vi "File Page - Get Log File Settings.vi"(7 "File Ctl Refs":T1, 8 "error in (no error)":errorcluster, 11 "Item Ref in":T11 format="%.0x") -> (0 "error out":errorcluster, 3 "Item Ref out":T11 format="%.0x")   [LabVIEW 2015, in "Waveform Data Logger System Explorer.lvlib"]
uses:
  Waveform Data Logger System Explorer.lvlib
  <vilib>/NI Veristand/Custom Device API/Custom Device Item Ref.ctl
  Types/File Ctl Refs.ctl
  Types/File - Spec Ctl Refs.ctl
  Types/File - Wfm Ctl Refs.ctl
  Types/File - Settings Ctl Refs.ctl
  Shared/Classes/Log File Specifications/Log File Specification/File Conflict Operation.ctl
  Types/File - Start Trig Ctl Refs.ctl
  Shared/Types/Start Trigger.ctl
  Shared/Types/Default Trigger.ctl
  Shared/Types/Digital Trigger.ctl
  Shared/Types/Analog Trigger.ctl
  Shared/Types/In Range Trigger.ctl
  Shared/Types/Value Change Trigger.ctl
  Shared/Types/Boolean Trigger.ctl
  Types/Single Node Browser Data.ctl
  <vilib>/NI Veristand/UI Controls/Single Node Browser/Single Node Browser Ref.ctl
  NationalInstruments.VeriStand.SystemStorageUI
  <vilib>/NI Veristand/UI Controls/Single Node Browser/Callback Type.ctl
  <vilib>/NI Veristand/UI Controls/Single Node Browser/Net Event Data.ctl
  <vilib>/NI Veristand/UI Controls/Single Node Browser/Net Event.ctl
  Types/File - Stop Trig Ctl Refs.ctl
  Shared/Types/Stop Trigger.ctl
  Types/File - Advanced Ctl Refs.ctl
  Types/Log Timestamps.ctl
  Shared/Globals/Property Strings.vi
  <vilib>/NI Veristand/Custom Device API/Get Item Property (Boolean).vi
  <vilib>/NI Veristand/Custom Device API/Get Item Property (String).vi
  <vilib>/NI Veristand/Custom Device API/Get Item Property (U16).vi
  <vilib>/NI Veristand/Custom Device API/Get Item Property (Double).vi
  Shared/Waveform Data Logger Shared.lvlib
  <vilib>/NI VeriStand/Custom Device API/Custom Device API.lvlib
  Shared/Classes/Log File Specifications/Log File Specification/Log File Specification.lvclass
  <vilib>/NI VeriStand/UI Controls/Single Node Browser/NI_VS UI Single Node Browser.lvlib
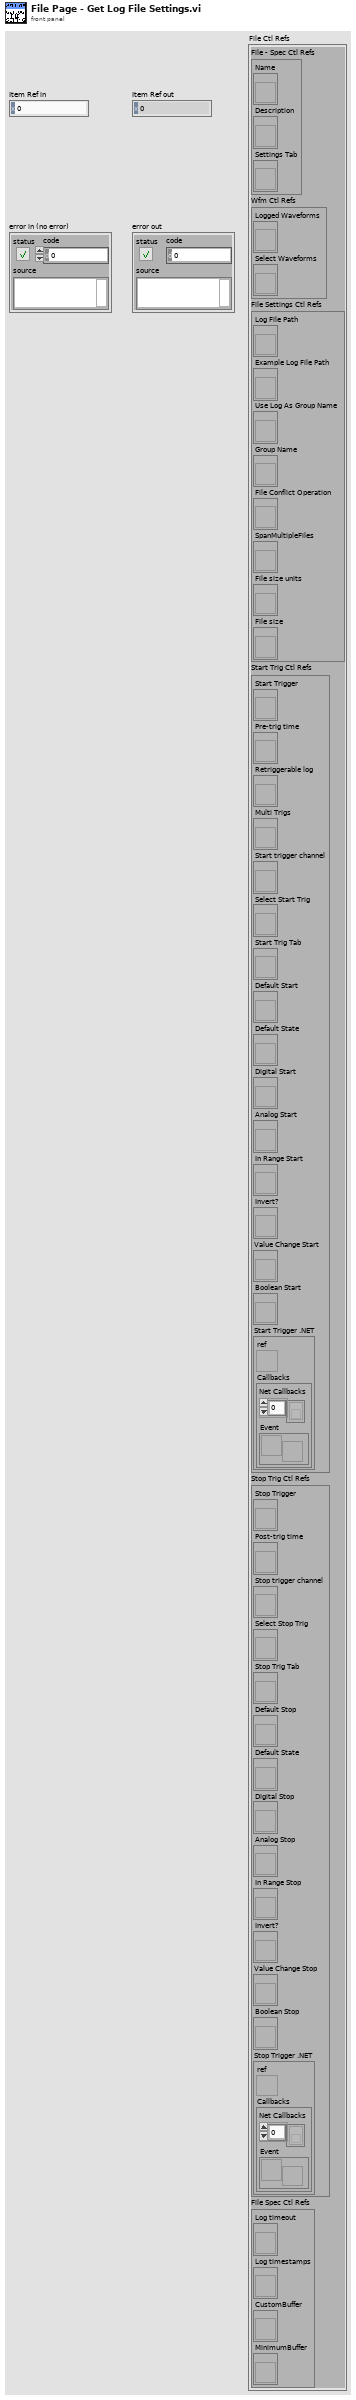
[diagram p1: front panel]
types:
  T1 = typedef "Waveform Data Logger System Explorer.lvlib/File Ctl Refs.ctl" = cluster{"File Spec Ctl Refs":T2, "Wfm Ctl Refs":T3, "File Settings Ctl Refs":T4, "Start Trig Ctl Refs":T5, "Stop Trig Ctl Refs":T9, "File Spec Ctl Refs":T10}
  T2 = typedef "Waveform Data Logger System Explorer.lvlib/File - Spec Ctl Refs.ctl" = cluster{"Name":refnum<vi>, "Description":refnum<vi>, "Settings Tab":refnum<vi>}
  T3 = typedef "Waveform Data Logger System Explorer.lvlib/File - Wfm Ctl Refs.ctl" = cluster{"Logged Waveforms":refnum<vi>, "Select Waveforms":refnum<vi>}
  T4 = typedef "Waveform Data Logger System Explorer.lvlib/File - Settings Ctl Refs.ctl" = cluster{"Log File Path":refnum<vi>, "Example Log File Path":refnum<vi>, "Use Log As Group Name":refnum<vi>, "Group Name":refnum<vi>, "File Conflict Operation":refnum<vi>, "SpanMultipleFiles":refnum<vi>, "File size units":refnum<vi>, "File size":refnum<vi>}
  T5 = typedef "Waveform Data Logger System Explorer.lvlib/File - Start Trig Ctl Refs.ctl" = cluster{"Start Trigger":refnum<vi>, "Pre-trig time":refnum<vi>, "Retriggerable log":refnum<vi>, "Multi Trigs":refnum<vi>, "Start trigger channel":refnum<vi>, "Select Start Trig":refnum<vi>, "Start Trig Tab":refnum<vi>, "Default Start":refnum<vi>, "Default State":refnum<vi>, "Digital Start":refnum<vi>, "Analog Start":refnum<vi>, "In Range Start":refnum<vi>, "Invert?":refnum<vi>, "Value Change Start":refnum<vi>, "Boolean Start":refnum<vi>, "Start Trigger .NET":T6}
  T6 = typedef "Waveform Data Logger System Explorer.lvlib/Single Node Browser Data.ctl" = cluster{"ref":T7, "Callbacks":T8}
  T7 = typedef "NI_VS UI Single Node Browser.lvlib/Single Node Browser Ref.ctl" = refnum<k24>
  T8 = typedef "NI_VS UI Single Node Browser.lvlib/Callback Type.ctl" = cluster{"Net Callbacks":refnum<k27>[], "Event":refnum<user-event>}
  T9 = typedef "Waveform Data Logger System Explorer.lvlib/File - Stop Trig Ctl Refs.ctl" = cluster{"Stop Trigger":refnum<vi>, "Post-trig time":refnum<vi>, "Stop trigger channel":refnum<vi>, "Select Stop Trig":refnum<vi>, "Stop Trig Tab":refnum<vi>, "Default Stop":refnum<vi>, "Default State":refnum<vi>, "Digital Stop":refnum<vi>, "Analog Stop":refnum<vi>, "In Range Stop":refnum<vi>, "Invert?":refnum<vi>, "Value Change Stop":refnum<vi>, "Boolean Stop":refnum<vi>, "Stop Trigger .NET":T6}
  T10 = typedef "Waveform Data Logger System Explorer.lvlib/File - Advanced Ctl Refs.ctl" = cluster{"Log timeout":refnum<vi>, "Log timestamps":refnum<vi>, "CustomBuffer":refnum<vi>, "MinimumBuffer":refnum<vi>}
  T11 = typedef "Custom Device API.lvlib/Custom Device Item Ref.ctl" = u64
  T12 = enum8{"Enabled", "Disabled", "Disabled and Grayed Out"}
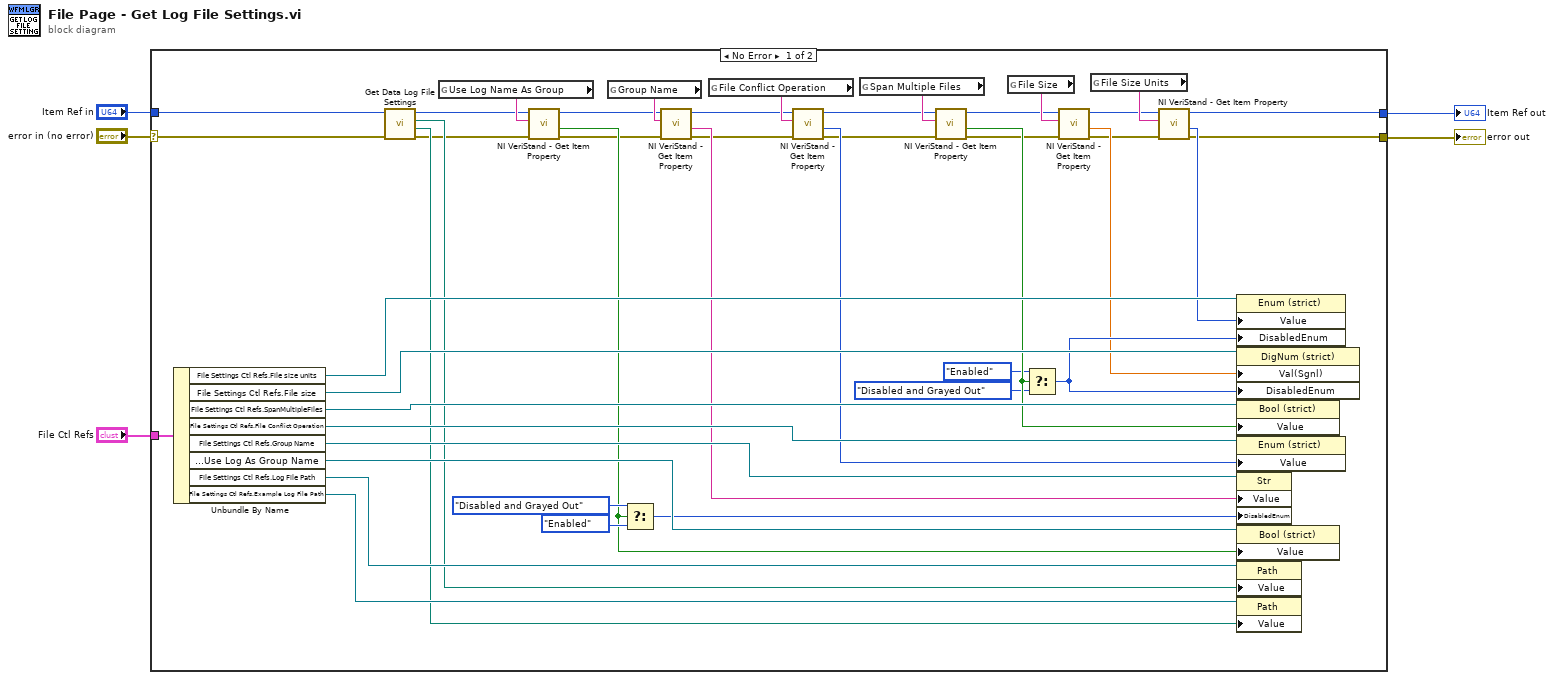
[diagram p0: block diagram]
diagram:
  n1 = case shown="No Error" "error in (no error)" {
    selector: "error in (no error)" -> [w40 w51]
    tunnel: [w9 w52] -> w5
    tunnel: [w8 w51] -> w4
    tunnel: "Item Ref in" -> [w41 w52]
    tunnel: "File Ctl Refs" -> [w50 _]
    frame No Error {
      n2 = Unbundle By Name(w50) -> ("File Settings Ctl Refs.File size units"=w42:refnum<vi>, "File Settings Ctl Refs.File size"=w43:refnum<vi>, "File Settings Ctl Refs.SpanMultipleFiles"=w44:refnum<vi>, "File Settings Ctl Refs.File Conflict Operation"=w45:refnum<vi>, "File Settings Ctl Refs.Group Name"=w46:refnum<vi>, "File Settings Ctl Refs.Use Log As Group Name"=w47:refnum<vi>, "File Settings Ctl Refs.Log File Path"=w48:refnum<vi>, "File Settings Ctl Refs.Example Log File Path"=w49:refnum<vi>)
      n3 = call "Get Data Log File Settings.vi"("error in"=w40, "File Ref in"=w41) -> ("error out"=w35:errorcluster, "Example File Path"=w39:path, "Log File Path"=w38:path, "File Ref out"=w36:T11)  [unwired: 6 out]
      n4 = global read "Property Strings.vi" "Use Log Name As Group"() -> (w37:string)
      n5 = call-poly <vilib>:"NI VeriStand - Get Item Property.vi"("error in (no error)"=w35, "Property Name"=w37, "Item Ref in"=w36) -> ("error out"=w28:errorcluster, "Value"=w31:bool, "Item Ref out"=w29:T11)  [unwired: 1 in, 5 out]
      n6 = global read "Property Strings.vi" "Group Name"() -> (w30:string)
      n7 = Select(t=T12."Disabled and Grayed Out" ("Disabled"), s=w31, f=T12."Enabled" ("Disabled")) -> (s? t:f=w32:T12)
      n8 = call-poly <vilib>:"NI VeriStand - Get Item Property.vi"("error in (no error)"=w28, "Property Name"=w30, "Item Ref in"=w29) -> ("error out"=w24:errorcluster, "Value"=w27:string, "Item Ref out"=w25:T11)  [unwired: 1 in, 5 out]
      n9 = global read "Property Strings.vi" "File Conflict Operation"() -> (w26:string)
      n10 = call-poly <vilib>:"NI VeriStand - Get Item Property.vi"("error in (no error)"=w24, "Property Name"=w26, "Item Ref in"=w25) -> ("error out"=w20:errorcluster, "Value"=w23:u16, "Item Ref out"=w21:T11)  [unwired: 1 in, 5 out]
      n11 = global read "Property Strings.vi" "Span Multiple Files"() -> (w22:string)
      n12 = call-poly <vilib>:"NI VeriStand - Get Item Property.vi"("error in (no error)"=w20, "Property Name"=w22, "Item Ref in"=w21) -> ("error out"=w15:errorcluster, "Value"=w18:bool, "Item Ref out"=w16:T11)  [unwired: 1 in, 5 out]
      n13 = global read "Property Strings.vi" "File Size"() -> (w17:string)
      n14 = Select(t=T12."Enabled" ("Disabled"), s=w18, f=T12."Disabled and Grayed Out" ("Disabled")) -> (s? t:f=w19:T12)
      n15 = call-poly <vilib>:"NI VeriStand - Get Item Property.vi"("error in (no error)"=w15, "Property Name"=w17, "Item Ref in"=w16) -> ("error out"=w11:errorcluster, "Value"=w14:dbl, "Item Ref out"=w12:T11)  [unwired: 1 in, 5 out]
      n16 = global read "Property Strings.vi" "File Size Units"() -> (w13:string)
      n17 = call-poly <vilib>:"NI VeriStand - Get Item Property.vi"("error in (no error)"=w11, "Property Name"=w13, "Item Ref in"=w12) -> ("error out"=w8:errorcluster, "Value"=w10:u16, "Item Ref out"=w9:T11)  [unwired: 1 in, 5 out]
      n18 = property on="Property Node" class="Enum (strict)"(reference=w42, "Value"=w10, "DisabledEnum"=w19) -> ()  [unwired: 1 in, 2 out]
      n19 = property on="Property Node" class="DigNum (strict)"(reference=w43, "Val(Sgnl)"=w14, "DisabledEnum"=w19) -> ()  [unwired: 1 in, 2 out]
      n20 = property class="Bool (strict)"(reference=w44, "Value"=w18) -> ()  [unwired: 1 in, 2 out]
      n21 = property class="Enum (strict)"(reference=w45, "Value"=w23) -> ()  [unwired: 1 in, 2 out]
      n22 = property class="Str"(reference=w46, "Value"=w27, "DisabledEnum"=w32) -> ()  [unwired: 1 in, 2 out]
      n23 = property class="Bool (strict)"(reference=w47, "Value"=w31) -> ()  [unwired: 1 in, 2 out]
      n24 = property class="Path"(reference=w48, "Value"=w38) -> ()  [unwired: 1 in, 2 out]
      n25 = property class="Path"(reference=w49, "Value"=w39) -> ()  [unwired: 1 in, 2 out]
    }
    frame Error {
    }
  }
  "error out" <- w4
  "Item Ref out" <- w5
